vi "GenericLinearSensorSubVI.vi"(1 "Raw Input":dbl, 2 "Offset":dbl, 3 "Slope":dbl) -> (0 "Scaled Output":dbl)   [LabVIEW 2016]
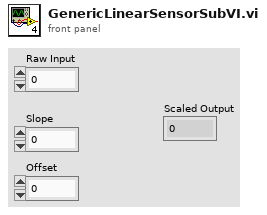
[diagram p1: front panel]
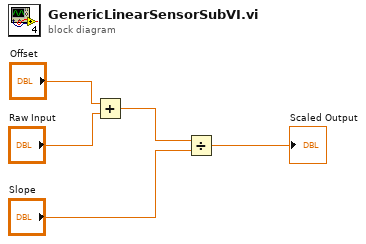
[diagram p0: block diagram]
diagram:
  n1 = Add(x="Offset", y="Raw Input") -> (x+y=w2:dbl)
  n2 = Divide(x=w2, y="Slope") -> (x/y=→"Scaled Output":dbl)
